vi "GetConfidence.vi"(9 "Measured Values":T1, 10 "Calib Coefficients":T1) -> (2 "Confidence":dbl)   [LabVIEW 2018, in "ColorSensor.lvlib"]
uses:
  ColorSensor.lvlib
  TypeDef/NormColorValues.ctl
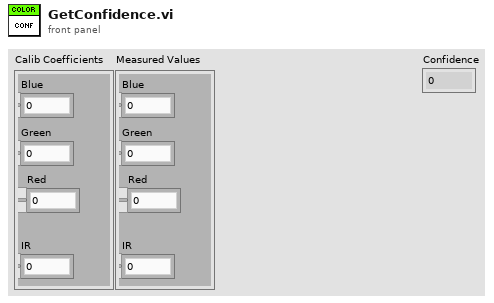
[diagram p1: front panel]
types:
  T1 = typedef "ColorSensor.lvlib/NormColorValues.ctl" = cluster{"Blue":dbl, "Green":dbl, "Red":dbl, "IR":dbl}
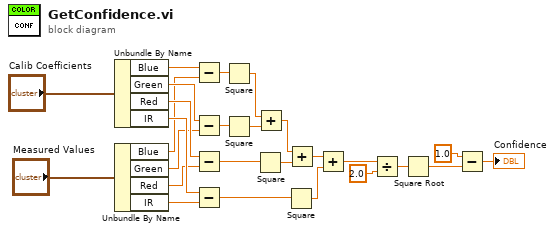
[diagram p0: block diagram]
diagram:
  n1 = Unbundle By Name("Calib Coefficients") -> ("Blue"=w24:dbl, "Green"=w23:dbl, "Red"=w22:dbl, "IR"=w21:dbl)
  n2 = Unbundle By Name("Measured Values") -> ("Blue"=w20:dbl, "Green"=w19:dbl, "Red"=w18:dbl, "IR"=w17:dbl)
  n3 = Subtract(x=w24, y=w20) -> (x-y=w16:dbl)
  n4 = Subtract(x=w23, y=w19) -> (x-y=w15:dbl)
  n5 = Subtract(x=w22, y=w18) -> (x-y=w14:dbl)
  n6 = Subtract(x=w21, y=w17) -> (x-y=w13:dbl)
  n7 = Square(x=w16) -> (x^2=w12:dbl)
  n8 = Square(x=w15) -> (x^2=w11:dbl)
  n9 = Square(x=w14) -> (x^2=w9:dbl)
  n10 = Add(x=w12, y=w11) -> (x+y=w10:dbl)
  n11 = Square(x=w13) -> (x^2=w7:dbl)
  n12 = Add(x=w10, y=w9) -> (x+y=w8:dbl)
  n13 = Add(x=w8, y=w7) -> (x+y=w6:dbl)
  n14 = Divide(x=w6, y=2.0) -> (x/y=w2:dbl)
  n15 = Square Root(x=w2) -> (sqrt(x)=w1:dbl)
  n16 = Subtract(x=1.0, y=w1) -> (x-y=→"Confidence":dbl)
